vi "palindrome_word.vi"(0 "Word":string, 7 "check":bool) -> ()   [LabVIEW 2020]
doc: "Checks if an entered word is palindrome or not."
panel:
  out "Palindrome or not":bool
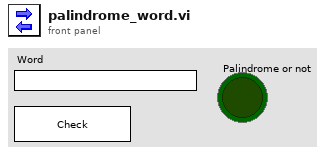
[diagram p1: front panel]
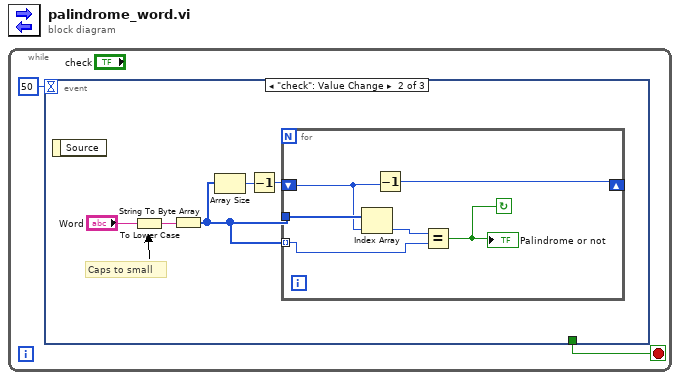
[diagram p0: block diagram]
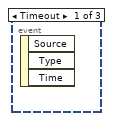
[diagram p2: hidden frame]
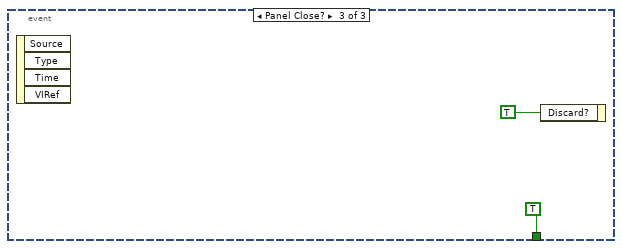
[diagram p3: hidden frame]
diagram:
  n1 = while {
    stop <- w1 stop-if-true
    n2 = event shown="[1] \"check\": Value Change" {
      selector: _ -> [_ _ _]
      dyn-events: _ -> [_ _ _]
      timeout: 50 -> [_ _ _]
      tunnel: [_ _ TRUE] -> w1
      event Timeout {
        n3 = event-data() -> ()  [unwired: 1 in, 3 out]
      }
      event "check": Value Change {
        # "Caps to small"
        n4 = event-data() -> ()  [unwired: 1 in, 1 out]
        n5 = To Lower Case(string="Word") -> (all lower case string=w3:string)
        n6 = String To Byte Array(string=w3) -> (unsigned byte array=w7:u8[])
        n7 = Array Size(array=w7) -> (size(s)=w5:i32)
        n8 = Decrement(x=w5) -> (x-1=w6:i32)
        n9 = for {
          tunnel: w7 -> [w13]
          shift-right: [w12] -> _
          shift-left: w6 -> [w11]
          tunnel: w7 -> [w9] mode=indexing
          stop <- w8 continue-if-true
          n10 = Index Array(array=w13, index=w11) -> (element=w10:u8)
          n11 = Decrement(x=w11) -> (x-1=w12:i32)
          n12 = Equal?(x=w10, y=w9) -> (x = y?=w8:bool)
          "Palindrome or not" <- w8
        }
      }
      event Panel Close? {
        n13 = event-data() -> ()  [unwired: 1 in, 4 out]
        n14 = event-data("Discard?"=TRUE) -> ()  [unwired: 1 in, 1 out]
      }
    }
  }
